vi "全加器电路实验.vi"() -> ()   [LabVIEW 2018]
panel:
  in  "结束":bool
  out "进位C":bool
  out "和数":bool
  in  "低位进位C1":bool
  in  "加数B":bool
  in  "被加数A":bool
  # "74HC00：与非门"
  # "74HC20：四输入与非门"
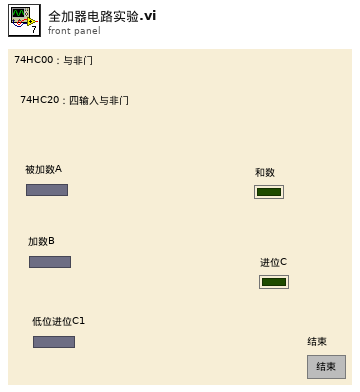
[diagram p1: front panel]
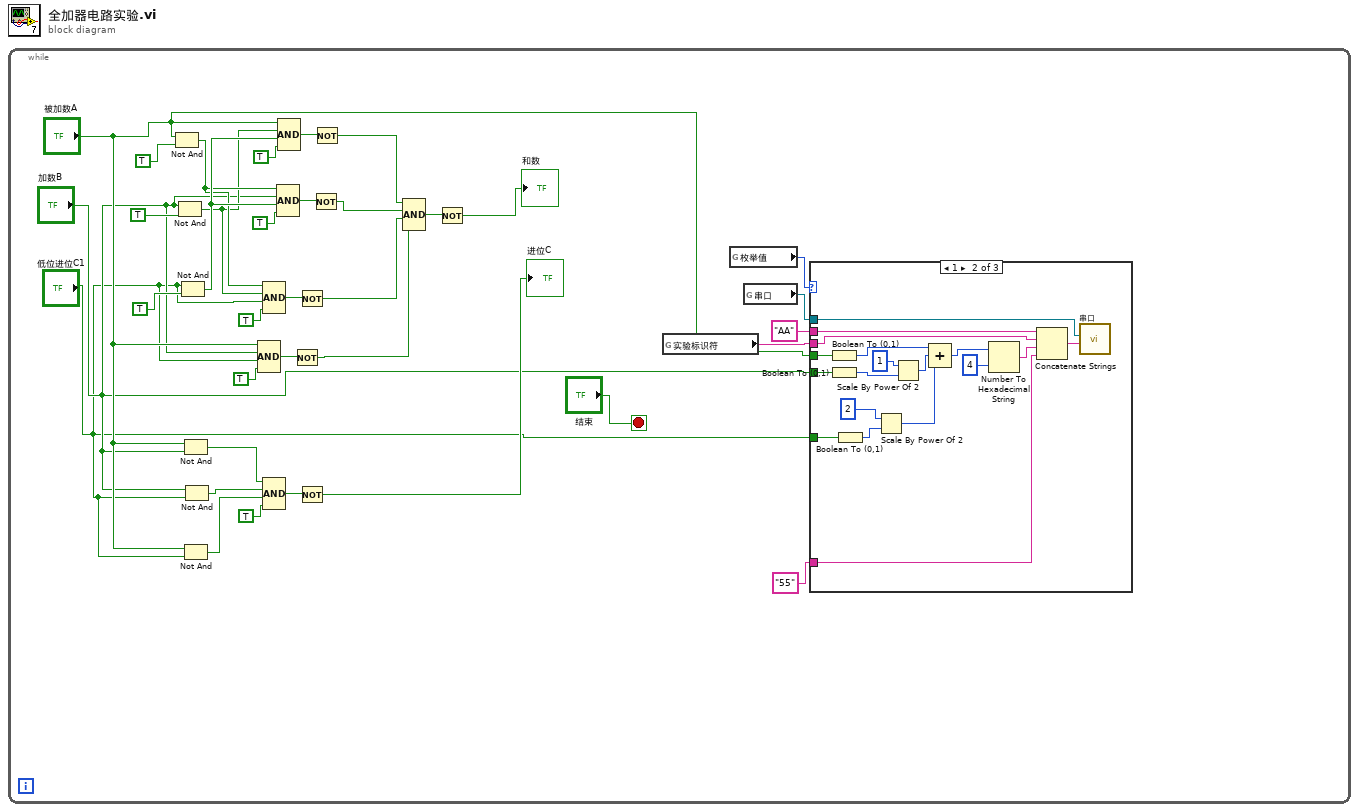
[diagram p0: block diagram]
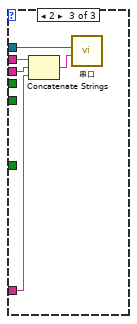
[diagram p3: hidden frame]
diagram:
  n1 = while {
    stop <- "结束" stop-if-true
    n2 = Not And(1:TRUE, 2:"被加数A") -> (0:w17:bool)
    n3 = Not And(1:TRUE, 2:"加数B") -> (0:w16:bool)
    n4 = Not And(1:TRUE, 2:"低位进位C1") -> (0:w18:bool)
    n5 = Not And(1:"加数B", 2:"被加数A") -> (0:w12:bool)
    n6 = Not And(1:"低位进位C1", 2:"被加数A") -> (0:w10:bool)
    n7 = Not And(1:"低位进位C1", 2:"加数B") -> (0:w11:bool)
    n8 = Compound Arithmetic op=AND ("复合运算")("被加数A", "加数B", "低位进位C1", TRUE) -> (w27:bool)
    n9 = Compound Arithmetic op=AND ("复合运算")(w17, w16, "低位进位C1", TRUE) -> (w29:bool)
    n10 = Compound Arithmetic op=AND ("复合运算")(w12, w11, w10, TRUE) -> (w13:bool)
    n11 = Compound Arithmetic op=AND ("复合运算")(w17, "加数B", w18, TRUE) -> (w31:bool)
    n12 = Compound Arithmetic op=AND ("复合运算")("被加数A", w16, w18, TRUE) -> (w33:bool)
    n13 = Not(x=w27) -> (.not. x?=w22:bool)
    n14 = Not(x=w29) -> (.not. x?=w23:bool)
    n15 = Not(x=w13) -> (.not. x?=→"进位C":bool)
    n16 = Not(x=w31) -> (.not. x?=w24:bool)
    n17 = Not(x=w33) -> (.not. x?=w25:bool)
    n18 = Compound Arithmetic op=AND ("复合运算")(w25, w24, w23, w22) -> (w26:bool)
    n19 = Not(x=w26) -> (.not. x?=→"和数":bool)
    n20 = global read "全局变量.vi" "实验标识符"() -> (w6:string)
    n21 = global read "全局变量.vi" "枚举值"() -> (w8:i8)
    n22 = global read "全局变量.vi" "串口"() -> (w7:refnum<visa-resource-name>)
    n23 = case shown="1" w8 {
      tunnel: "加数B" -> [_ w48 _]
      tunnel: "被加数A" -> [_ w47 _]
      tunnel: w7 -> [_ w46 w56]
      tunnel: w6 -> [_ w45 w57]
      tunnel: "55" -> [_ w44 w54]
      tunnel: "AA" -> [_ w43 w55]
      tunnel: "低位进位C1" -> [_ w37 _]
      frame 0, Default {
      }
      frame 1 {
        n24 = Boolean To (0,1)(Boolean=w47) -> (0, 1=w52:i16)
        n25 = Boolean To (0,1)(Boolean=w48) -> (0, 1=w50:i16)
        n26 = Boolean To (0,1)(Boolean=w37) -> (0, 1=w38:i16)
        n27 = Scale By Power Of 2(n=2, x=w38) -> (x*2^n=w39:i16)
        n28 = Scale By Power Of 2(n=1, x=w50) -> (x*2^n=w51:i16)
        n29 = Compound Arithmetic op=ADD ("复合运算")(w52, w51, w39) -> (w42:i16)
        n30 = Number To Hexadecimal String(1:4, 2:w42) -> (0:w40:string)
        n31 = Concatenate Strings(w43, w45, w40, w44) -> (w53:string)
        n32 = call "串口.vi"("字符串"=w53, "VISA resource name"=w46) -> ()  [unwired: 10 in]
      }
      frame 2 {
        n33 = Concatenate Strings(w55, w57, w54) -> (w58:string)
        n34 = call "串口.vi"("字符串"=w58, "VISA resource name"=w56) -> ()  [unwired: 10 in]
      }
    }
  }
